vi "KM_ControlHFLI -- fast -- V2.vi"(4 "Control HFLI command":T2=enum."Scan frequency", 8 "ZI HFLI System Parameters IN":T1={"IP Address"="DEV987", "Start (Hz)"=10000.0, "Stop (Hz)"=1000000.0, "Filter Order"=4, "Number of Points"=100, "Precision"=0, "Bandwidth (Hz)"=-1.0, "Averaging"=1, "Log Sweep"=FALSE, "Demod"=3} {"Averaging" items=["1"=1, "2"=2, "4"=4, "16"=16, "32"=32, "64"=64]; "Bandwidth (Hz)" format="%#_p"; "Precision" items=["Low", "Med", "High"]; "Number of Points" min=2 max=66000; "Filter Order" items=["6, 1st"=1, "12, 2nd"=2, "18, 3rd"=3, "24, 4th"=4, "30, 5th"=5, "36, 6th"=6, "42, 7th"=7, "48, 8th"=8]; "Stop (Hz)" format="%_5p"; "Start (Hz)" format="%_5p"}) -> (0 "Voltage out":cdb[](array[numeric]), 1 "Freq out":dbl[](array[numeric]), 3 "ZI HFLI System Parameters OUT":T1={"IP Address"="DEV987", "Start (Hz)"=10000.0, "Stop (Hz)"=1000000.0, "Filter Order"=4, "Number of Points"=100, "Precision"=0, "Bandwidth (Hz)"=-1.0, "Averaging"=1, "Log Sweep"=FALSE, "Demod"=3} {"Averaging" items=["1"=1, "2"=2, "4"=4, "16"=16, "32"=32, "64"=64]; "Bandwidth (Hz)" format="%#_p"; "Precision" items=["Low", "Med", "High"]; "Number of Points" min=2 max=66000; "Filter Order" items=["6, 1st"=1, "12, 2nd"=2, "18, 3rd"=3, "24, 4th"=4, "30, 5th"=5, "36, 6th"=6, "42, 7th"=7, "48, 8th"=8]; "Stop (Hz)" format="%_5p"; "Start (Hz)" format="%_5p"})   [LabVIEW 2015]
doc: "Control a Zurich instrument device via the LabOne Labview API. \nRequirements: Zurich Instruments HF2 (HF2IS or HF2LI-MF ).\nThis example uses the API functions to perform a frequency sweep and measure the impedance. \n\n© Zurich Instruments AG, www.zhinst.com"
uses:
  Zurich/Zurich Instruments/LabOne/API/LabVIEW/Zurich Instruments LabOne/Zurich Instruments LabOne.lvlib
  KM_ControlHFLIcommand.ctl
  KM_SystemParameters.ctl
panel:
  out "cal_types":cluster{string[], bool[]}[](array[cluster])=[{["R (Ohms)", " ", " "], [TRUE, FALSE, FALSE]}, {["C (F)", " ", " "], [TRUE, FALSE, FALSE]}, {["L (H)", " ", " "], [TRUE, FALSE, FALSE]}, {["R (Ohms)", "C (F)\n ", " "], [TRUE, TRUE, FALSE]}]
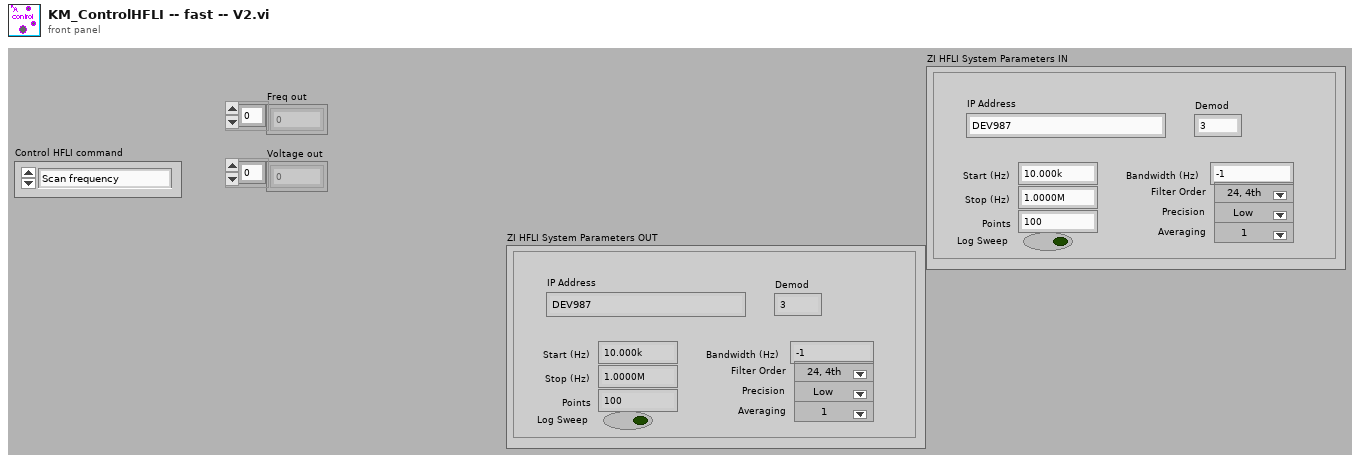
[diagram p1: front panel]
types:
  T1 = typedef "KM_SystemParameters.ctl" = cluster{"IP Address":string, "Start (Hz)":dbl, "Stop (Hz)":dbl, "Filter Order":i32, "Number of Points":i32, "Precision":u16, "Bandwidth (Hz)":dbl, "Averaging":u16, "Log Sweep":bool, "Demod":i32}
  T2 = typedef "KM_ControlHFLIcommand.ctl" = enum16{"Initialize", "Scan frequency"}
  T3 = typedef "Zurich Instruments LabOne.lvlib/ziTypeHandle.ctl" = cluster{"handleValid":bool, "Conn":u64, "Path Prefix":string, "Handle":u64, "Connected":bool, "Clockbase(s)":dbl}
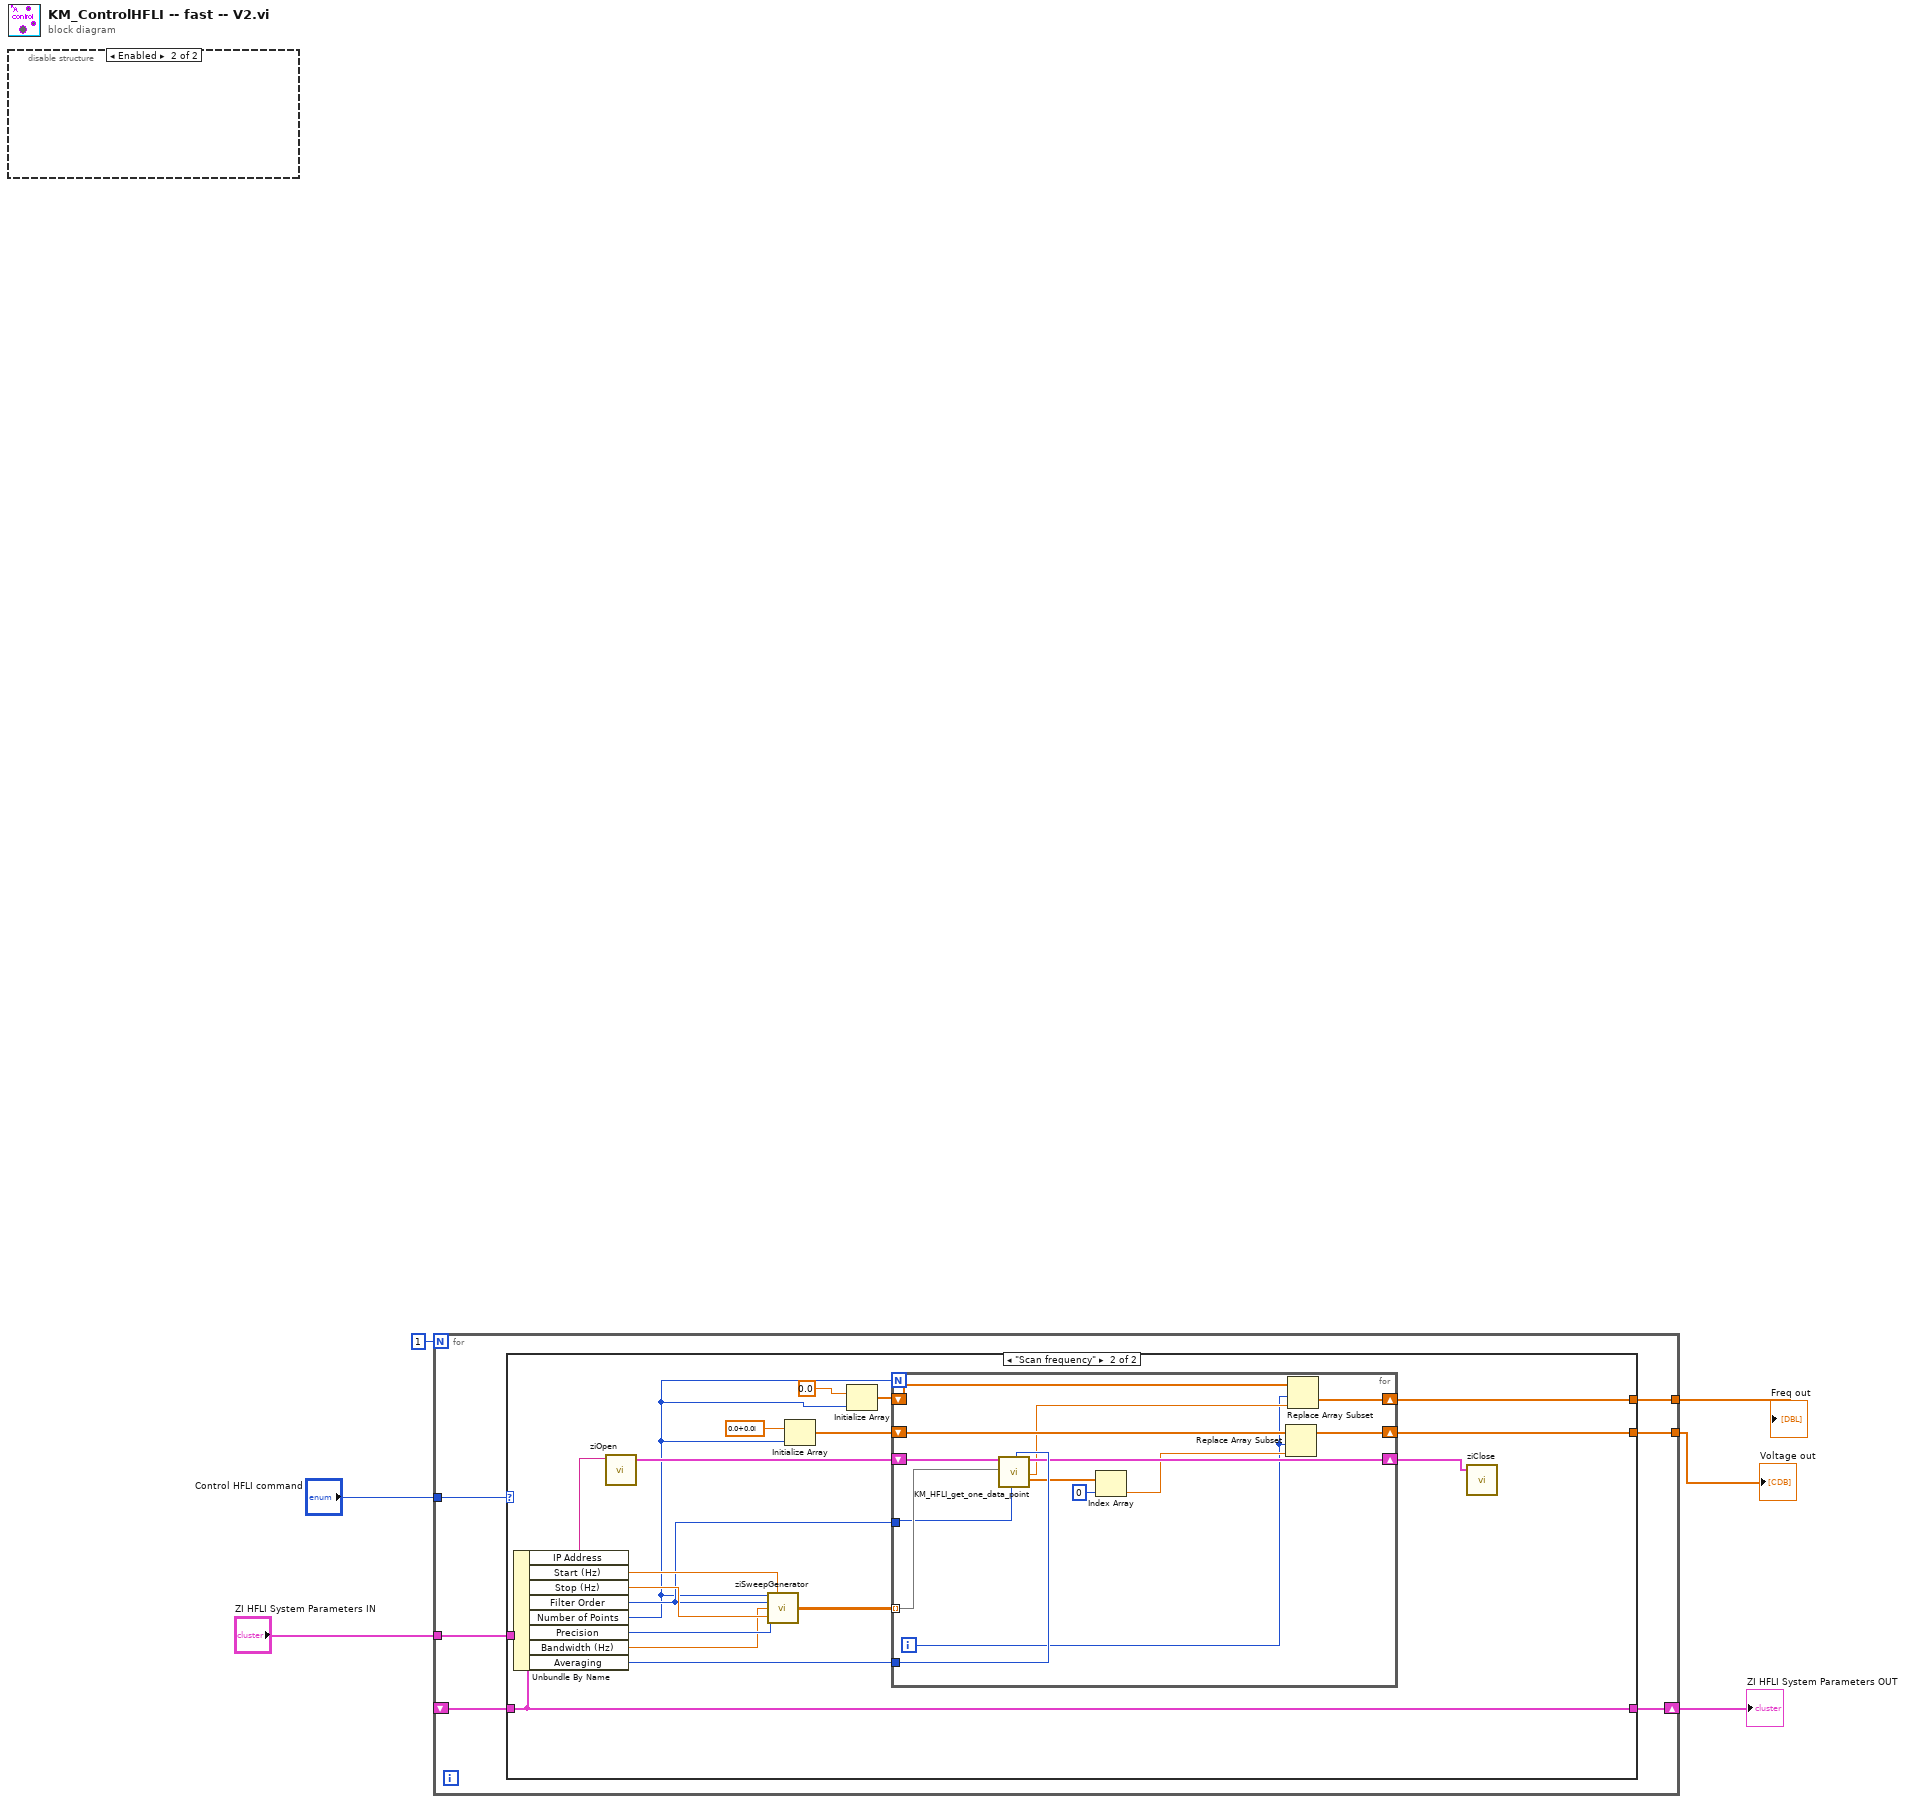
[diagram p0: block diagram]
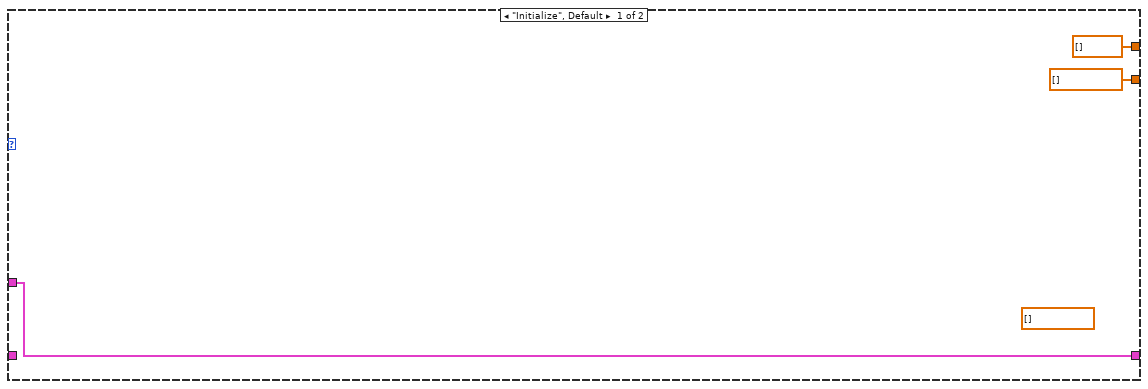
[diagram p2: hidden frame]
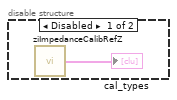
[diagram p3: hidden frame]
diagram:
  n1 = disable-structure shown="Enabled" {
    frame Disabled {
      n2 = call "ziImpedanceCalibRefZ.vi"() -> ("cal_types"=→"cal_types":cluster{string[], bool[]}[], 2:w7)  [unwired: 3 in, 1 out]
    }
    frame Enabled {
    }
  }
  n3 = for {
    N: 1 -> [_]
    tunnel: "Control HFLI command" -> [w14]
    tunnel: "ZI HFLI System Parameters IN" -> [w13]
    shift-right: [w12] -> w2
    shift-left: _ -> [w11]
    tunnel: [w10] -> w4
    tunnel: [w9] -> w3
    n4 = case shown="\"Scan frequency\"" w14 {
      tunnel: w13 -> [w17 _]
      tunnel: [w17 w35] -> w12
      tunnel: w11 -> [_ w35]
      tunnel: [dbl[] [] w20] -> w10
      tunnel: [cdb[] [] w19] -> w9
      frame "Initialize", Default {
        (unwired) cdb[] []
      }
      frame "Scan frequency" {
        n5 = Unbundle By Name(w35) -> ("IP Address"=w34:string, "Start (Hz)"=w33:dbl, "Stop (Hz)"=w32:dbl, "Filter Order"=w26:i32, "Number of Points"=w18:i32, "Precision"=w31:u16, "Bandwidth (Hz)"=w30:dbl, "Averaging"=w25:u16)
        n6 = call "ziOpen.vi"("Address"=w34) -> ("HandleOut"=w22:T3)  [unwired: 3 in, 2 out]
        n7 = call "ziSweepGenerator.vi"("Steps (#)"=w18, "Start (Hz)"=w33, "Order (4)"=w26, "Bandwith (-1=auto)"=w30, "Precision (Low)"=w31, "Stop (Hz)"=w32) -> ("Sweep Sequence (F (Hz), BW (Hz), TC(s), Time(s))"=w27:dbl[][])  [unwired: 7 in, 2 out]
        n8 = Initialize Array(cdb 0.0+0.0i ("element"), w18) -> (w28:cdb[])
        n9 = Initialize Array(0.0 ("element"), w18) -> (w23:dbl[])
        n10 = for {
          N: w18 -> [_]
          shift-right: [w48] -> w19
          shift-left: w28 -> [w49]
          tunnel: w26 -> [w40]
          tunnel: w25 -> [w47]
          shift-right: [w45] -> w20
          shift-left: w23 -> [w46]
          shift-right: [w44] -> w21
          shift-left: w22 -> [w43]
          tunnel: w27 -> [w42] mode=indexing
          i -> [w36]
          n11 = call "KM_HFLI_get_one_data_point.vi"("Handle In"=w43, "Freq Sequence In"=w42, "Order (4)"=w40, "Averaging"=w47) -> ("Handle Out"=w44:T3, "Frequency OUT"=w41:dbl, "z OUT"=w39:cdb[])  [unwired: 12 in, 1 out]
          n12 = Index Array(array=w39, index=0) -> (element=w37:cdb)
          n13 = Replace Array Subset(array=w49, new element=w37, index=w36) -> (w48:cdb[])
          n14 = Replace Array Subset(array=w46, new element=w41, index=w36) -> (w45:dbl[])
        }
        n15 = call "ziClose.vi"("Handle In"=w21) -> ()  [unwired: 3 in, 2 out]
      }
    }
  }
  "Freq out" <- w4
  "Voltage out" <- w3
  "ZI HFLI System Parameters OUT" <- w2
